vi "Timeout Watchdog.vi"(11 "Buffered Log Sink in":refnum<class "Buffered String Log Sink.lvclass">) -> ()   [LabVIEW 2018, in "MVA Framework.lvlib" / "Buffered String Log Sink.lvclass"]
uses:
  Buffered String Log Sink.lvclass
  String Log Sink/String Log Sink.lvclass
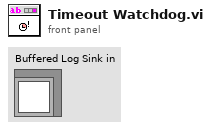
[diagram p1: front panel]
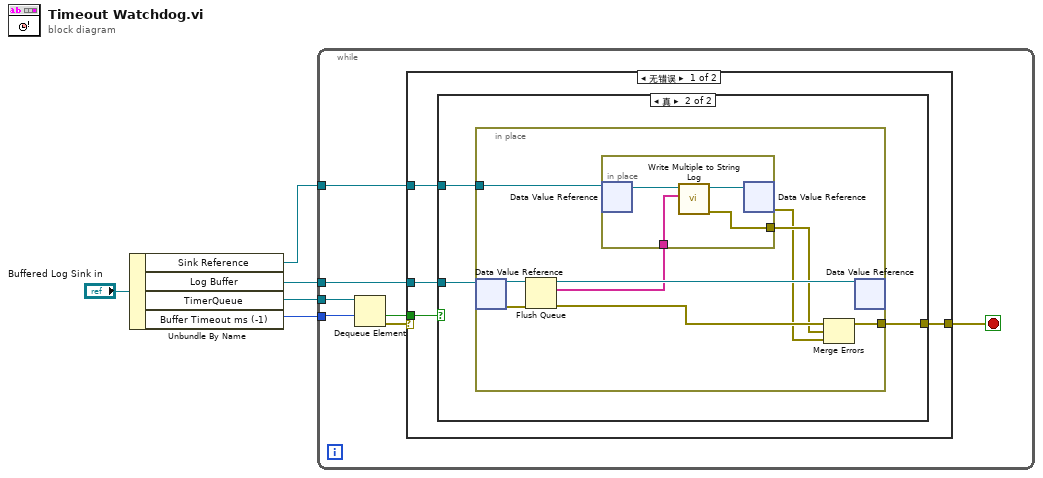
[diagram p0: block diagram]
diagram:
  n1 = Unbundle By Name("Buffered Log Sink in") -> ("Sink Reference"=w1:refnum<data-value>, "Log Buffer"=w4:refnum<data-value>, "TimerQueue"=w3:refnum<queue>, "Buffer Timeout ms (-1)"=w2:i32)
  n2 = while {
    tunnel: w4 -> [w8]
    tunnel: w3 -> [w12]
    tunnel: w2 -> [w11]
    tunnel: w1 -> [w7]
    stop <- w6 stop-if-true
    n3 = Dequeue Element(queue=w12, timeout in ms (-1)=w11) -> (timed out?=w9:bool, error out=w10:errorcluster)  [unwired: 1 in, 2 out]
    n4 = case shown="无错误" w10 {
      selector: w10 -> [_ w33]
      tunnel: w9 -> [w16 _]
      tunnel: w8 -> [w15 _]
      tunnel: w7 -> [w14 _]
      tunnel: [w13 w33] -> w6
      frame No Error {
        n5 = case shown="真" w16 {
          tunnel: w15 -> [_ w19]
          tunnel: w14 -> [_ w17]
          tunnel: [_ w18] -> w13
          frame False {
          }
          frame True {
            n6 = in-place {
              in-place-border: [w24] -> w18
              in-place-border: w17 -> [w23]
              n7 = in-place-dvr #1(w19) -> (w28:refnum<queue>, w27:errorcluster)
              n8 = Flush Queue(queue=w28, error in (no error)=w27) -> (queue out=w25:refnum<queue>, remaining elements=w20:string[], error out=w26:errorcluster)
              n9 = in-place {
                in-place-border: [w30] -> w22
                in-place-border: w20 -> [w29]
                n10 = in-place-dvr #2(w23) -> (w32:refnum<class "String Log Sink.lvclass">)  [unwired: 1 out]
                n11 = call-dynamic "Write Multiple to String Log.vi"("Strings to Log"=w29, "String Log Sink in"=w32) -> ("error out"=w30:errorcluster, "String Log Sink out"=w31:refnum<class "String Log Sink.lvclass">)  [unwired: 8 in]
                n12 = in-place-dvr #2(w31) -> (w21:errorcluster)  [unwired: 1 out]
              }
              n13 = Merge Errors(w26, w22, w21) -> (w24:errorcluster)
              n14 = in-place-dvr #1(w25) -> ()  [unwired: 2 out]
            }
          }
        }
      }
      frame Error {
      }
    }
  }
